vi "Receiver.Test.vi"() -> ()   [LabVIEW 2016]
uses:
  <vilib>/Distrio/LabbitMQ/Connection/Connection.lvclass
  <vilib>/Distrio/LabbitMQ/Channel/queue_declare_cluster.ctl
  <vilib>/Distrio/LabbitMQ/Connection/connection_parameters_cluster.ctl
  <vilib>/Distrio/LabbitMQ/Channel/exchange_type_enum.ctl
  global/AMQP_credentials.vi
  <vilib>/Distrio/LabbitMQ/Channel/Channel.lvclass
  <vilib>/Distrio/LabbitMQ/Queue/Queue.lvclass
panel:
  out "stopLoop":bool
  in  "STOPbutton":bool
  out "error out":errorcluster
  out "consumer: received message":string
  in  "binding key":string[](array[string])=["broadcast.#"]
  in  "QueueDeclare Properties":T1={"queue"="AMQP_test", "durable (F)"=FALSE, "exclusive (F)"=TRUE, "autoDelete (F)"=FALSE, "561934e089]], mscorlib, Version=0.0.0.0, Culture=neutral, PublicKeyToken=b77a5c561934e089\targuments"=refnum}
  in  "error (in)":errorcluster
  in  "host name":string="higgsino.physics.ucsb.edu"
  in  "Connection in":refnum<class "Connection.lvclass">
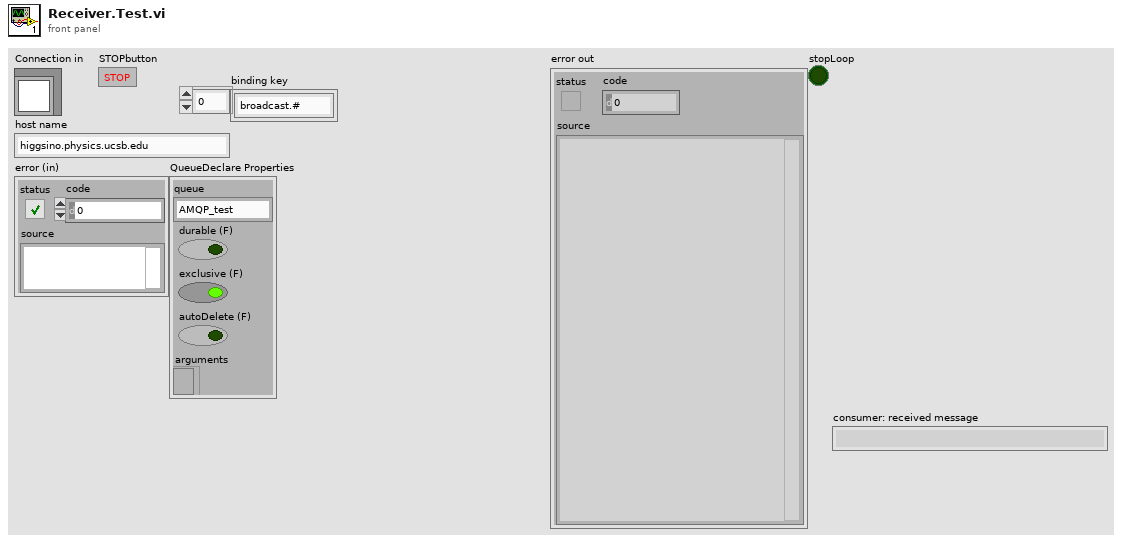
[diagram p1: front panel]
types:
  T1 = typedef "Channel.lvclass/queue_declare_cluster.ctl" = cluster{"queue":string, "durable (F)":bool, "exclusive (F)":bool, "autoDelete (F)":bool, "561934e089]], mscorlib, Version=0.0.0.0, Culture=neutral, PublicKeyToken=b77a5c561934e089\targuments":refnum<k24>}
  T2 = typedef "Connection.lvclass/connection_parameters_cluster.ctl" = cluster{"host name":string, "port":i32, "user name":string, "password":string, "virtual host":string}
  T3 = typedef "Channel.lvclass/exchange_type_enum.ctl" = enum16{"direct", "topic", "fanout", "headers"}
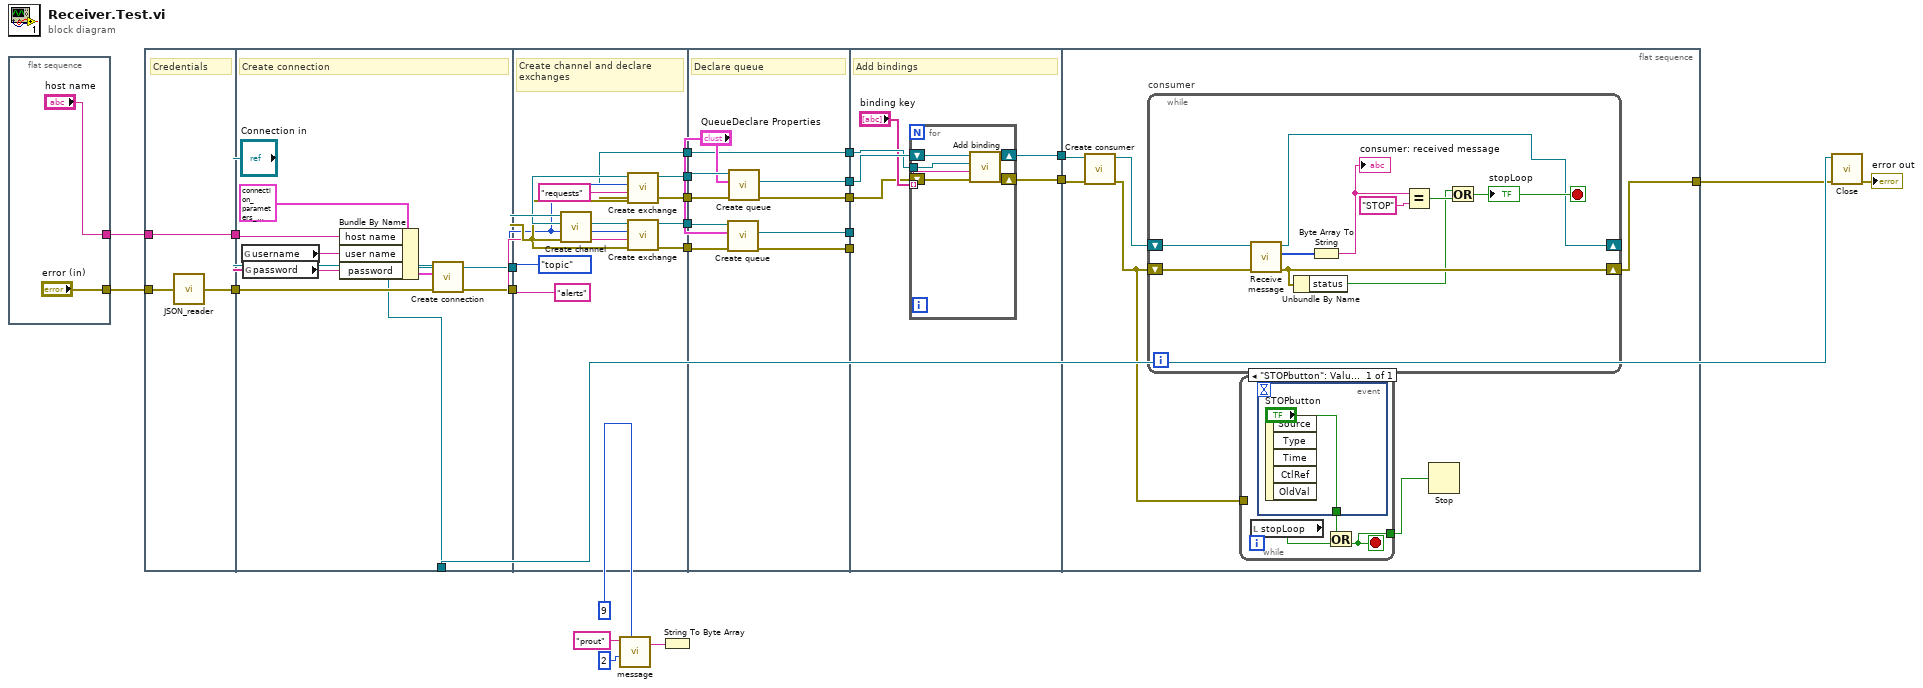
[diagram p0: block diagram]
diagram:
  n1 = flat-sequence {
    tunnel: ["error (in)"] -> w23
    tunnel: ["host name"] -> w22
    frame #0 {
    }
  }
  n2 = flat-sequence {
    tunnel: [w28] -> w25
    tunnel: [w30] -> w24
    tunnel: w23 -> [w29]
    tunnel: w22 -> [w28]
    tunnel: w25 -> [w34]
    tunnel: w24 -> [w33]
    tunnel: [w31] -> w21
    tunnel: [w32] -> w20
    tunnel: [w31] -> w3
    tunnel: w21 -> [w51]
    tunnel: w20 -> [w50]
    tunnel: [w44] -> w15
    tunnel: [w43] -> w14
    tunnel: [w42] -> w13
    tunnel: [w41] -> w12
    tunnel: [w40] -> w6
    tunnel: w15 -> [w61]
    tunnel: w14 -> [w60]
    tunnel: w13 -> [w57]
    tunnel: w12 -> [w56]
    tunnel: [w59] -> w11
    tunnel: [w58] -> w10
    tunnel: [w54] -> w9
    tunnel: [w53] -> w8
    tunnel: [w52] -> w7
    tunnel: w6 -> [w52]
    tunnel: w11 -> [_]
    tunnel: w10 -> [_]
    tunnel: w9 -> [w62]
    tunnel: w8 -> [w67]
    tunnel: w7 -> [w66]
    tunnel: [w64] -> w5
    tunnel: [w63] -> w4
    tunnel: w5 -> [w78]
    tunnel: w4 -> [w77]
    tunnel: [w76] -> w2
    frame #0 {
      # "Credentials"
      n3 = call "JSON_reader.vi"("error (in)"=w29) -> ("error (out)"=w30:errorcluster)
    }
    frame #1 {
      # "Create connection"
      n4 = global read "AMQP_credentials.vi" "username"() -> (w36:string)
      n5 = global read "AMQP_credentials.vi" "password"() -> (w35:string)
      n6 = Bundle By Name(cluster=T2 {"host name"="localhost", "port"=5672, "user name"="guest", "password"="guest", "virtual host"="/"} ("connection parameters"), "host name"=w34, "user name"=w36, "password"=w35) -> (w37:T2)
      n7 = call <vilib>:"Create connection.vi"("error in (no error)"=w33, "connection parameters"=w37, "Connection in"="Connection in") -> ("error out"=w32:errorcluster, "Connection out"=w31:refnum<class "Connection.lvclass">)  [unwired: 7 in]
    }
    frame #2 {
      w45 = exchange_type_enum."topic" ("exchange type")
      # "Create channel and declare exchanges"
      n8 = call <vilib>:"Create channel.vi"("error in (no error)"=w50, "Connection in"=w51) -> ("error out"=w46:errorcluster, "channel"=w48:refnum<class "Channel.lvclass">)  [unwired: 7 in, 1 out]
      n9 = call <vilib>:"Create exchange.vi"("error in (no error)"=w46, "exchange name"="requests", "exchange type"=w45, "Channel in"=w48) -> ("error out"=w41:errorcluster, "Exchange.lvclass"=w40:refnum<class "Exchange.lvclass">, "Channel out"=w42:refnum<class "Channel.lvclass">)  [unwired: 5 in]
      n10 = call <vilib>:"Create exchange.vi"("error in (no error)"=w46, "exchange name"="alerts", "exchange type"=w45, "Channel in"=w48) -> ("error out"=w43:errorcluster, "Channel out"=w44:refnum<class "Channel.lvclass">)  [unwired: 5 in, 1 out]
    }
    frame #3 {
      # "Declare queue"
      n11 = call <vilib>:"Create queue.vi"("error in (no error)"=w60, "QueueDeclare Properties"="QueueDeclare Properties", "Channel in"=w61) -> ("error out"=w58:errorcluster, "Queue.lvclass"=w59:refnum<class "Queue.lvclass">)  [unwired: 6 in, 1 out]
      n12 = call <vilib>:"Create queue.vi"("error in (no error)"=w56, "QueueDeclare Properties"="QueueDeclare Properties", "Channel in"=w57) -> ("error out"=w54:errorcluster, "Queue.lvclass"=w53:refnum<class "Queue.lvclass">)  [unwired: 6 in, 1 out]
    }
    frame #4 {
      # "Add bindings"
      n13 = for {
        tunnel: w66 -> [w72]
        tunnel: "binding key" -> [w71] mode=indexing
        shift-right: [w70] -> w64
        shift-left: w67 -> [w73]
        shift-right: [w69] -> w63
        shift-left: w62 -> [w68]
        n14 = call <vilib>:"Add binding.vi"("error in (no error)"=w68, "binding key"=w71, "Exchange.lvclass"=w72, "Consumer in"=w73) -> ("error out"=w69:errorcluster, "Consumer out"=w70:refnum<class "Queue.lvclass">)  [unwired: 6 in]
      }
    }
    frame #5 {
      n15 = call <vilib>:"Create consumer.vi"("error in (no error)"=w77, "Queue in"=w78) -> ("error out"=w75:errorcluster, "Queue out"=w79:refnum<class "Queue.lvclass">)  [unwired: 8 in]
      n16 = while "consumer" {
        shift-right: [w91] -> w76
        shift-left: w75 -> [w93]
        shift-right: [w89] -> _
        shift-left: w79 -> [w92]
        stop <- w90 stop-if-true
        n17 = call <vilib>:"Receive message.vi"("error in (no error)"=w93, "Consumer in"=w92) -> ("error out"=w91:errorcluster, "message body"=w88:u8[], "Consumer out"=w89:refnum<class "Queue.lvclass">)  [unwired: 4 in, 3 out]
        n18 = Unbundle By Name(w91) -> ("status"=w84:bool)
        n19 = Byte Array To String(unsigned byte array=w88) -> (string=w87:string)
        "consumer: received message" <- w87
        n20 = Equal?(x=w87, y="STOP") -> (x = y?=w85:bool)
        n21 = Or(x=w84, y=w85) -> (x .or. y?=w90:bool)
        "stopLoop" <- w90
      }
      n22 = while {
        tunnel: w75 -> [_]
        tunnel: [w80] -> w74
        stop <- w80 stop-if-true
        n23 = local read "stopLoop"() -> (w82:bool)
        n24 = event shown="[0] \"STOPbutton\": Value Change" {
          selector: _ -> [_]
          dyn-events: _ -> [_]
          timeout: _ -> [_]
          tunnel: ["STOPbutton"] -> w81
          event "STOPbutton": Value Change {
            n25 = event-data() -> ()  [unwired: 1 in, 5 out]
          }
        }
        n26 = Or(x=w81, y=w82) -> (x .or. y?=w80:bool)
      }
      n27 = Stop(stop? (T)=w74) -> ()
    }
  }
  n28 = call "message.vi"("msgop"=9, "msgtype"=2, "input"="prout") -> ("body"=w16:string)  [unwired: 3 in, 1 out]
  n29 = String To Byte Array(string=w16) -> ()  [unwired: 1 out]
  n30 = call <vilib>:"Close.vi"("error in (no error)"=w2, "Connection in"=w3) -> ("error out"=→"error out":errorcluster)  [unwired: 8 in, 1 out]
